vi "IoT_CheckHandle.vi"(11 "Handle in":u32) -> (2 "Good Handle?":bool, 3 "Refnum out":T1)   [LabVIEW 2016]
uses:
  <vilib>/httpClient/ClientHandle.ctl
  <vilib>/httpClient/LabVIEWHTTPClient.lvlib
panel:
  out "headers":string
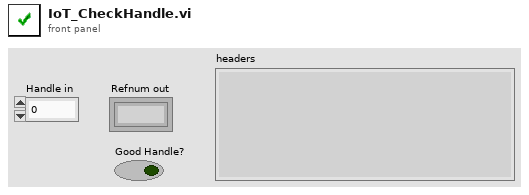
[diagram p1: front panel]
types:
  T1 = typedef "LabVIEWHTTPClient.lvlib/ClientHandle.ctl" = refnum<k1>
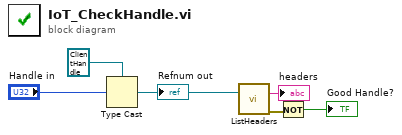
[diagram p0: block diagram]
diagram:
  n1 = Type Cast(type=T1 refnum ("Handle"), x="Handle in") -> (*(type *) &x=w4:T1)
  "Refnum out" <- w4
  n2 = call <vilib>:"ListHeaders.vi"("client handle"=w4) -> ("headers"=→"headers":string, "error out"=w3:errorcluster)  [unwired: 12 in, 1 out]
  n3 = Not(x=w3) -> (.not. x?=→"Good Handle?":bool)
